vi "Finish.vi"   [LabVIEW 2016]
doc: "This VI is called just before exiting. It is expected to close I/O refnum, save collected data, etc."
uses:
  <vilib>/Rock Robotics/WPI/Utilities/WPI_GetSetVariantRefNum.vi
types:
  T1 = typedef "WPI_SwitchDevRef.ctl" = cluster{"DevStatus":errorcluster, "DIO Channel":T2, "CntIndex":T3, "Normally Closed":bool}
  T2 = typedef "FPGA_DIOChannel.ctl" = enum8{"DIO 0", "DIO 1", "DIO 2", "DIO 3", "DIO 4", "DIO 5", "DIO 6", "DIO 7", "DIO 8", "DIO 9", "DIO MXP 0", "DIO MXP 1", "DIO MXP 2", "DIO MXP 3", "DIO MXP 4", "DIO MXP 5", "DIO MXP 6", "DIO MXP 7", "DIO MXP 8", "DIO MXP 9", "DIO MXP 10", "DIO MXP 11", "DIO MXP 12", "DIO MXP 13", "DIO MXP 14", "DIO MXP 15", "SPI Port CS1", "SPI Port CS2", "SPI Port CS3", "SPI Port MISO", "SPI Port MOSI", "Invalid"}
  T3 = typedef "FPGA_CounterCtrSystemIndex.ctl" = enum8{"Ctr 0", "Ctr 1", "Ctr 2", "Ctr 3", "Ctr 4", "Ctr 5", "Ctr 6", "Ctr 7", "Invalid"}
  T4 = typedef "WPI_DigitalOutputDevRef.ctl" = cluster{"DIO Channel":T2, "DevStatus":errorcluster}
  T5 = typedef "WPI_SolenoidDevRef.ctl" = cluster{"DevStatus":errorcluster, "Pneumatics Control Module":u8, "Forward Solenoid Channel":T6, "Reverse Solenoid Channel":T6}
  T6 = typedef "WPI_SolenoidChannel.ctl" = enum8{"Solenoid 0", "Solenoid 1", "Solenoid 2", "Solenoid 3", "Solenoid 4", "Solenoid 5", "Solenoid 6", "Solenoid 7", "Invalid"}
  T7 = typedef "WPI_MotorControlDeviceRef.ctl" = cluster{"DeviceStatus":errorcluster, "Type":T8, "PWM":cluster{"PWM Channel":T9, "DeadBand":T10}, "CAN":cluster{"Device Number":u8, "SetOutput VI Ref":variant, "GetOutput VI Ref":variant, "Enable VI Ref":variant, "Disable VI Ref":variant, "Data":variant}, "Invert":bool}
  T8 = typedef "WPI_MotorControlType.ctl" = enum16{"PWM", "CAN"}
  T9 = typedef "FPGA_DIOPWMChannel.ctl" = enum8{"PWM 0", "PWM 1", "PWM 2", "PWM 3", "PWM 4", "PWM 5", "PWM 6", "PWM 7", "PWM 8", "PWM 9", "PWM MXP 0", "PWM MXP 1", "PWM MXP 2", "PWM MXP 3", "PWM MXP 4", "PWM MXP 5", "PWM MXP 6", "PWM MXP 7", "PWM MXP 8", "PWM MXP 9", "Invalid"}
  T10 = typedef "WPI_PWMDeadband.ctl" = cluster{"Name":string, "maxPositivePwm":i32, "minPositivePwm":i32, "centerPwm":i32, "maxNegativePwm":i32, "minNegativePwm":i32, "angularRange":u16}
  T11 = typedef "WPI_JoystickDevRef.ctl" = cluster{"Device":T12}
  T12 = typedef "WPI_JoystickDeviceEnum.ctl" = enum16{"USB 0", "USB 1", "USB 2", "USB 3", "USB 4", "USB 5"}
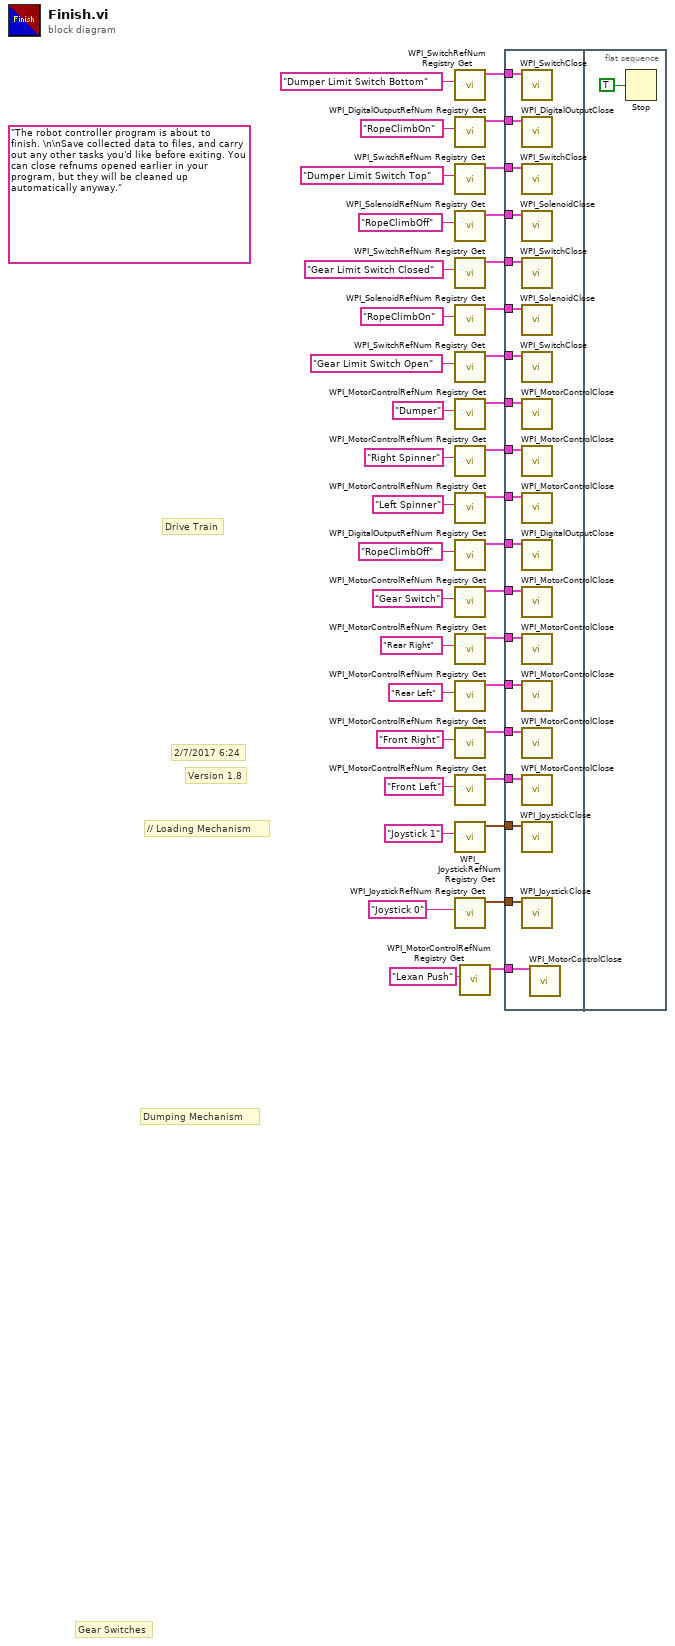
[diagram p0: block diagram]
diagram:
  (unwired) "The robot controller program is about to finish. \n\nSave collected data to files, and carry out any other tasks you'd like before exiting. You can close refnums opened earlier in your program, but they will be cleaned up automatically anyway."
  # "Gear Switches"
  # "Dumping Mechanism"
  # "Version 1.8"
  # "2/7/2017 6:24"
  # "Drive Train"
  # "// Loading Mechanism"
  n1 = call <vilib>:"WPI_SwitchRefNum Registry Get.vi"("refnum name"="Dumper Limit Switch Bottom") -> ("SwitchDevRef"=w3:T1)  [unwired: 9 in, 1 out]
  n2 = call <vilib>:"WPI_DigitalOutputRefNum Registry Get.vi"("refnum name"="RopeClimbOn") -> ("DigitalOutputDevRef"=w12:T4)  [unwired: 9 in, 1 out]
  n3 = call <vilib>:"WPI_SwitchRefNum Registry Get.vi"("refnum name"="Dumper Limit Switch Top") -> ("SwitchDevRef"=w13:T1)  [unwired: 9 in, 1 out]
  n4 = call <vilib>:"WPI_SolenoidRefNum Registry Get.vi"("refnum name"="RopeClimbOff") -> ("SolenoidDevRef"=w5:T5)  [unwired: 9 in, 1 out]
  n5 = call <vilib>:"WPI_SwitchRefNum Registry Get.vi"("refnum name"="Gear Limit Switch Closed") -> ("SwitchDevRef"=w17:T1)  [unwired: 9 in, 1 out]
  n6 = call <vilib>:"WPI_SolenoidRefNum Registry Get.vi"("refnum name"="RopeClimbOn") -> ("SolenoidDevRef"=w6:T5)  [unwired: 9 in, 1 out]
  n7 = call <vilib>:"WPI_SwitchRefNum Registry Get.vi"("refnum name"="Gear Limit Switch Open") -> ("SwitchDevRef"=w18:T1)  [unwired: 9 in, 1 out]
  n8 = call <vilib>:"WPI_MotorControlRefNum Registry Get.vi"("refnum name"="Dumper") -> ("MotorControlDevRef"=w22:T7)  [unwired: 9 in, 1 out]
  n9 = call <vilib>:"WPI_MotorControlRefNum Registry Get.vi"("refnum name"="Right Spinner") -> ("MotorControlDevRef"=w24:T7)  [unwired: 9 in, 1 out]
  n10 = call <vilib>:"WPI_MotorControlRefNum Registry Get.vi"("refnum name"="Left Spinner") -> ("MotorControlDevRef"=w23:T7)  [unwired: 9 in, 1 out]
  n11 = call <vilib>:"WPI_DigitalOutputRefNum Registry Get.vi"("refnum name"="RopeClimbOff") -> ("DigitalOutputDevRef"=w11:T4)  [unwired: 9 in, 1 out]
  n12 = call <vilib>:"WPI_MotorControlRefNum Registry Get.vi"("refnum name"="Gear Switch") -> ("MotorControlDevRef"=w20:T7)  [unwired: 9 in, 1 out]
  n13 = call <vilib>:"WPI_MotorControlRefNum Registry Get.vi"("refnum name"="Rear Right") -> ("MotorControlDevRef"=w33:T7)  [unwired: 9 in, 1 out]
  n14 = call <vilib>:"WPI_MotorControlRefNum Registry Get.vi"("refnum name"="Rear Left") -> ("MotorControlDevRef"=w34:T7)  [unwired: 9 in, 1 out]
  n15 = call <vilib>:"WPI_MotorControlRefNum Registry Get.vi"("refnum name"="Front Right") -> ("MotorControlDevRef"=w35:T7)  [unwired: 9 in, 1 out]
  n16 = call <vilib>:"WPI_MotorControlRefNum Registry Get.vi"("refnum name"="Front Left") -> ("MotorControlDevRef"=w36:T7)  [unwired: 9 in, 1 out]
  n17 = call <vilib>:"WPI_JoystickRefNum Registry Get.vi"("refnum name"="Joystick 1") -> ("JoystickDevRef"=w28:T11)  [unwired: 1 in, 9 out]
  n18 = call <vilib>:"WPI_JoystickRefNum Registry Get.vi"("refnum name"="Joystick 0") -> ("JoystickDevRef"=w37:T11)  [unwired: 1 in, 9 out]
  n19 = call <vilib>:"WPI_MotorControlRefNum Registry Get.vi"("refnum name"="Lexan Push") -> ("MotorControlDevRef"=w1:T7)  [unwired: 9 in, 1 out]
  n20 = flat-sequence {
    tunnel: w37 -> [w57]
    tunnel: w36 -> [w56]
    tunnel: w35 -> [w55]
    tunnel: w34 -> [w54]
    tunnel: w33 -> [w53]
    tunnel: w28 -> [w52]
    tunnel: w24 -> [w51]
    tunnel: w23 -> [w50]
    tunnel: w22 -> [w49]
    tunnel: w20 -> [w48]
    tunnel: w18 -> [w47]
    tunnel: w17 -> [w46]
    tunnel: w13 -> [w45]
    tunnel: w12 -> [w43]
    tunnel: w11 -> [w44]
    tunnel: w6 -> [w41]
    tunnel: w5 -> [w42]
    tunnel: w3 -> [w40]
    tunnel: w1 -> [w39]
    frame #0 {
      n21 = call <vilib>:"WPI_SwitchClose.vi"("SwitchDevRef"=w40) -> ()  [unwired: 10 in, 1 out]
      n22 = call <vilib>:"WPI_DigitalOutputClose.vi"("DigitalOutputDevRef"=w43) -> ()  [unwired: 10 in, 1 out]
      n23 = call <vilib>:"WPI_SwitchClose.vi"("SwitchDevRef"=w45) -> ()  [unwired: 10 in, 1 out]
      n24 = call <vilib>:"WPI_SolenoidClose.vi"("SolenoidDevRef"=w42) -> ()  [unwired: 10 in, 1 out]
      n25 = call <vilib>:"WPI_SwitchClose.vi"("SwitchDevRef"=w46) -> ()  [unwired: 10 in, 1 out]
      n26 = call <vilib>:"WPI_SolenoidClose.vi"("SolenoidDevRef"=w41) -> ()  [unwired: 10 in, 1 out]
      n27 = call <vilib>:"WPI_SwitchClose.vi"("SwitchDevRef"=w47) -> ()  [unwired: 10 in, 1 out]
      n28 = call <vilib>:"WPI_MotorControlClose.vi"("MotorControlDevRef"=w49) -> ()  [unwired: 10 in, 1 out]
      n29 = call <vilib>:"WPI_MotorControlClose.vi"("MotorControlDevRef"=w51) -> ()  [unwired: 10 in, 1 out]
      n30 = call <vilib>:"WPI_MotorControlClose.vi"("MotorControlDevRef"=w50) -> ()  [unwired: 10 in, 1 out]
      n31 = call <vilib>:"WPI_DigitalOutputClose.vi"("DigitalOutputDevRef"=w44) -> ()  [unwired: 10 in, 1 out]
      n32 = call <vilib>:"WPI_MotorControlClose.vi"("MotorControlDevRef"=w48) -> ()  [unwired: 10 in, 1 out]
      n33 = call <vilib>:"WPI_MotorControlClose.vi"("MotorControlDevRef"=w53) -> ()  [unwired: 10 in, 1 out]
      n34 = call <vilib>:"WPI_MotorControlClose.vi"("MotorControlDevRef"=w54) -> ()  [unwired: 10 in, 1 out]
      n35 = call <vilib>:"WPI_MotorControlClose.vi"("MotorControlDevRef"=w55) -> ()  [unwired: 10 in, 1 out]
      n36 = call <vilib>:"WPI_MotorControlClose.vi"("MotorControlDevRef"=w56) -> ()  [unwired: 10 in, 1 out]
      n37 = call <vilib>:"WPI_JoystickClose.vi"("JoystickDevRef"=w52) -> ()  [unwired: 11 out]
      n38 = call <vilib>:"WPI_JoystickClose.vi"("JoystickDevRef"=w57) -> ()  [unwired: 11 out]
      n39 = call <vilib>:"WPI_MotorControlClose.vi"("MotorControlDevRef"=w39) -> ()  [unwired: 10 in, 1 out]
    }
    frame #1 {
      n40 = Stop(stop? (T)=TRUE ("Quit")) -> ()
    }
  }
